vi "FGV Dato.vi"(10 "Funcion":enum16{"Guardar", "Leer"}(ring), 11 "Dato In":dbl) -> (3 "Dato Out":dbl)   [LabVIEW 2019]
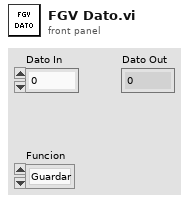
[diagram p1: front panel]
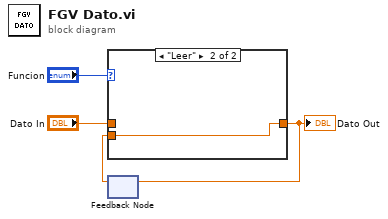
[diagram p0: block diagram]
diagram:
  n1 = feedback #1() -> (w2:dbl)  [unwired: 1 in]
  n2 = case shown="\"Leer\"" "Funcion" {
    tunnel: [w5 w6] -> w1
    tunnel: "Dato In" -> [w5 _]
    tunnel: w2 -> [_ w6]
    frame "Guardar", Default {
    }
    frame "Leer" {
    }
  }
  "Dato Out" <- w1
  n3 = feedback-in #1(w1) -> ()
